vi "sig_processing.vi"(8 "error in (no error)":errorcluster, 9 "Operation":T1, 11 "Input Data Cluster":T3) -> (0 "error out":errorcluster, 3 "Output Data":T2)   [LabVIEW 2018]
uses:
  <vilib>/Utility/file.llb/Read Delimited Spreadsheet (string).vi
  <vilib>/Utility/file.llb/Read Delimited Spreadsheet (DBL).vi
  sig_processing_data_cluster.ctl
  sig_proc_output_data.ctl
  sig_processing_state_defining_enum.ctl
panel:
  out "Note":string
  in  "NotesPath":path
  in  "FreqsPath":path
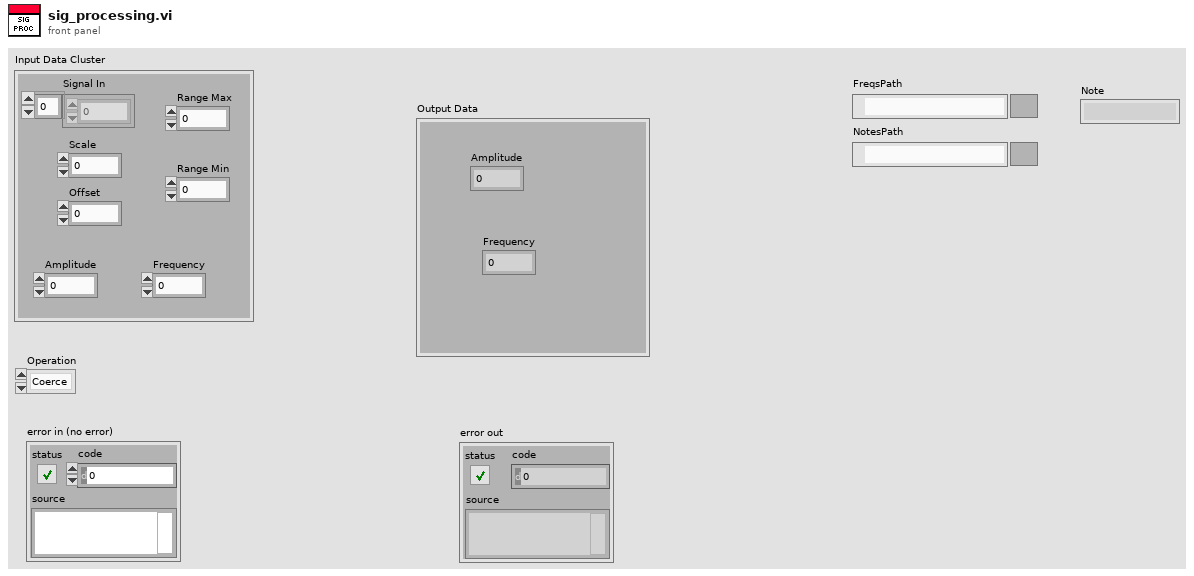
[diagram p1: front panel]
types:
  T1 = typedef "sig_processing_state_defining_enum.ctl" = enum16{"Coerce", "Scale", "Offset", "Norm"}
  T2 = typedef "sig_proc_output_data.ctl" = cluster{"Amplitude":dbl, "Frequency":dbl}
  T3 = typedef "sig_processing_data_cluster.ctl" = cluster{"Signal In":dbl[], "Scale":dbl, "Offset":dbl, "Range Max":dbl, "Range Min":dbl, "Amplitude":dbl, "Frequency":dbl}
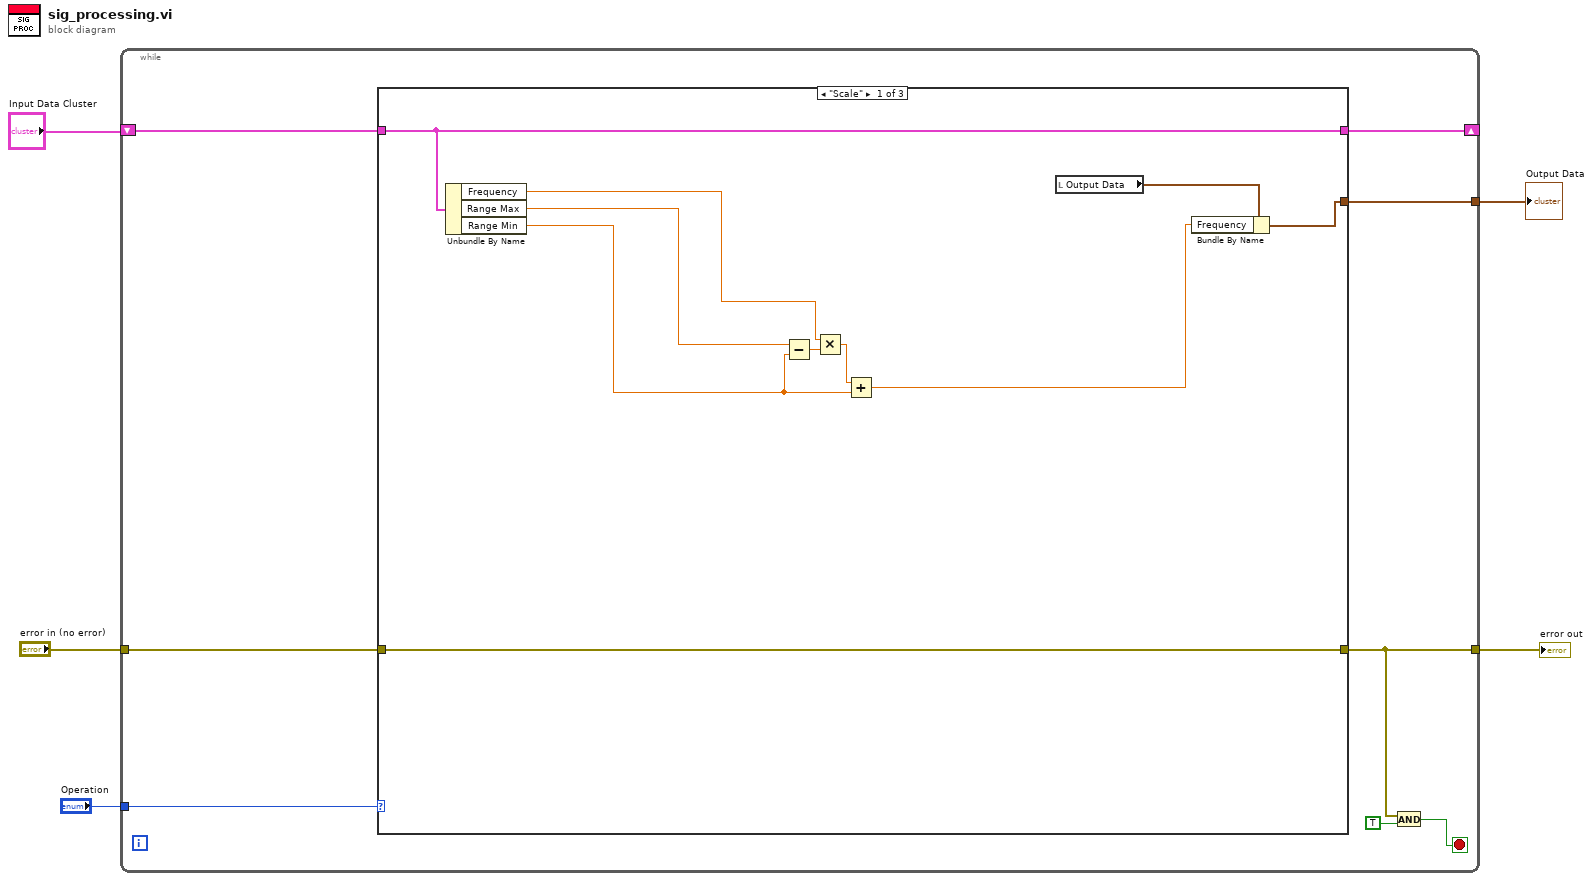
[diagram p0: block diagram]
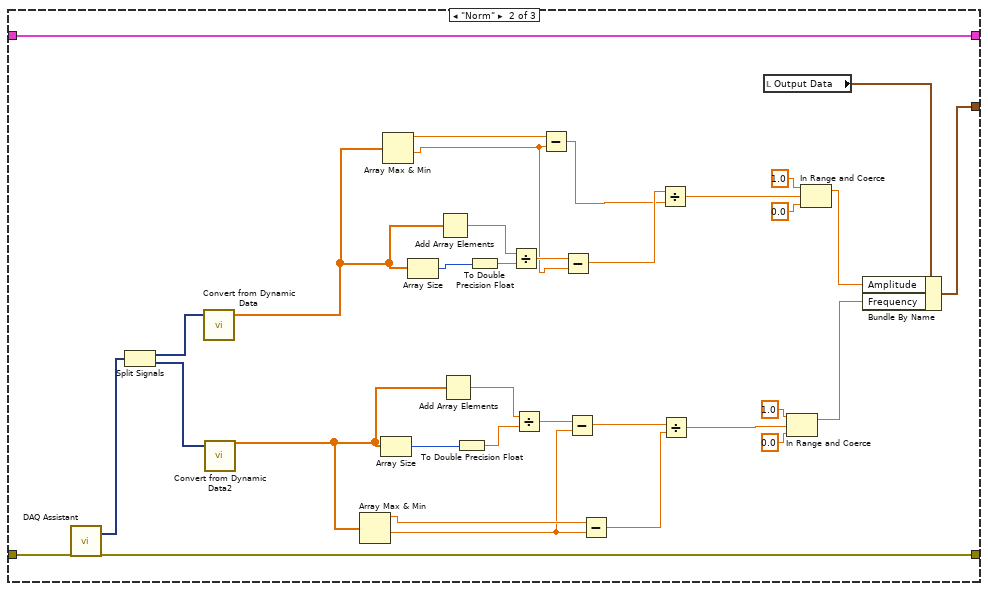
[diagram p2: hidden frame]
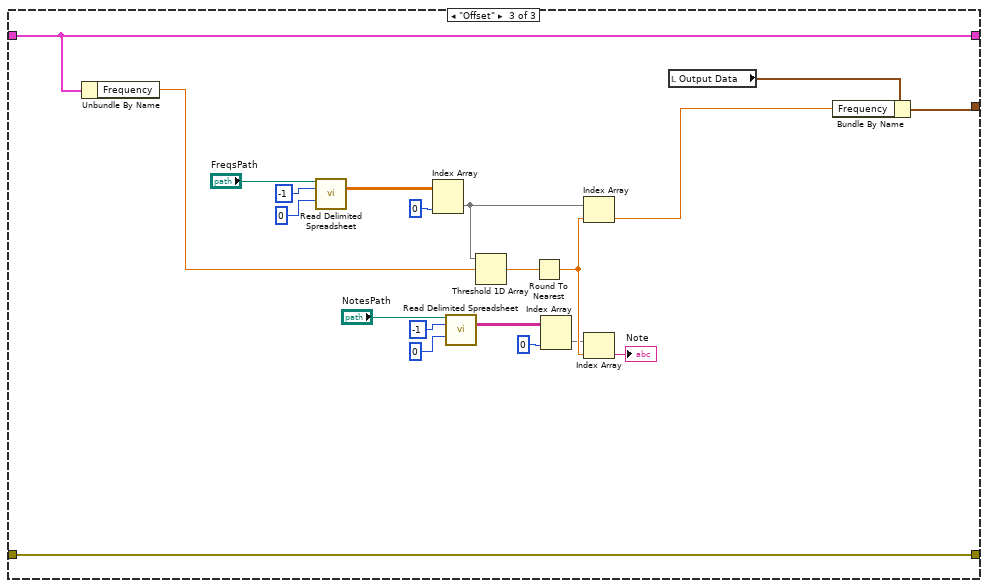
[diagram p3: hidden frame]
diagram:
  n1 = while {
    tunnel: "Operation" -> [w13]
    shift-right: [w10] -> _
    shift-left: "Input Data Cluster" -> [w11]
    tunnel: "error in (no error)" -> [w12]
    tunnel: [w8] -> w4
    tunnel: [w6] -> w2
    stop <- w7 stop-if-true
    n2 = case shown="\"Scale\"" w13 {
      tunnel: w12 -> [w23 w48 w78]
      tunnel: [w23 w47 w78] -> w8
      tunnel: w11 -> [w20 w42 w62]
      tunnel: [w20 w42 w62] -> w10
      tunnel: [w14 w33 w60] -> w6
      frame "Scale" {
        n3 = Unbundle By Name(w20) -> ("Frequency"=w19:dbl, "Range Max"=w18:dbl, "Range Min"=w17:dbl)
        n4 = Subtract(x=w18, y=w17) -> (x-y=w22:dbl)
        n5 = Multiply(x=w19, y=w22) -> (x*y=w21:dbl)
        n6 = Add(x=w21, y=w17) -> (x+y=w15:dbl)
        n7 = local read "Output Data"() -> (w16:T2)
        n8 = Bundle By Name(cluster=w16, "Frequency"=w15) -> (w14:T2)
      }
      frame "Norm" {
        n9 = call "DAQ Assistant"("error in"=w48) -> ("data"=w57:dynamicdata, "error out"=w47:errorcluster)  [unwired: 16 in, 1 out]
        n10 = Split Signals(w57) -> (w56:dynamicdata, w50:dynamicdata)  [unwired: 2 in]
        n11 = call "Convert from Dynamic Data"("Dynamic Data Type"=w56) -> ("Array"=w38:dbl[])  [unwired: 3 in]
        n12 = call "Convert from Dynamic Data2"("Dynamic Data Type"=w50) -> ("Array"=w37:dbl[])  [unwired: 3 in]
        n13 = Array Max & Min(array=w37) -> (max value=w36:dbl, min value=w34:dbl)  [unwired: 2 out]
        n14 = Array Size(array=w37) -> (size(s)=w51:i32)
        n15 = Array Max & Min(array=w38) -> (max value=w41:dbl, min value=w39:dbl)  [unwired: 2 out]
        n16 = Array Size(array=w38) -> (size(s)=w45:i32)
        n17 = Add Array Elements(numeric array=w38) -> (sum=w55:dbl)
        n18 = Add Array Elements(numeric array=w37) -> (sum=w52:dbl)
        n19 = To Double Precision Float(number=w51) -> (double precision float=w44:dbl)
        n20 = To Double Precision Float(number=w45) -> (double precision float=w46:dbl)
        n21 = Divide(x=w55, y=w46) -> (x/y=w54:dbl)
        n22 = Divide(x=w52, y=w44) -> (x/y=w49:dbl)
        n23 = Subtract(x=w41, y=w39) -> (x-y=w40:dbl)
        n24 = Subtract(x=w54, y=w39) -> (x-y=w53:dbl)
        n25 = Subtract(x=w49, y=w34) -> (x-y=w43:dbl)
        n26 = Subtract(x=w36, y=w34) -> (x-y=w35:dbl)
        n27 = Divide(x=w53, y=w40) -> (x/y=w25:dbl)
        n28 = Divide(x=w43, y=w35) -> (x/y=w29:dbl)
        n29 = local read "Output Data"() -> (w32:T2)
        n30 = In Range and Coerce(upper limit=1.0, x=w29, lower limit=0.0) -> (coerced(x)=w28:dbl)  [unwired: 1 out]
        n31 = In Range and Coerce(upper limit=1.0, x=w25, lower limit=0.0) -> (coerced(x)=w24:dbl)  [unwired: 1 out]
        n32 = Bundle By Name(cluster=w32, "Amplitude"=w24, "Frequency"=w28) -> (w33:T2)
      }
      frame "Offset" {
        n33 = Unbundle By Name(w62) -> ("Frequency"=w61:dbl)
        n34 = call-poly <vilib>:"Read Delimited Spreadsheet.vi"("file path (dialog if empty)"="FreqsPath", "number of rows (all:-1)"=-1, "max characters/row  (no limit:0)"=0) -> ("all rows"=w74:dbl[][])  [unwired: 7 in, 5 out]
        n35 = Index Array(array=w74, index (col)=0 ("index (row)")) -> (element=w66:dbl[])  [unwired: 1 in]
        n36 = call-poly <vilib>:"Read Delimited Spreadsheet.vi"("file path (dialog if empty)"="NotesPath", "number of rows (all:-1)"=-1, "max characters/row  (no limit:0)"=0) -> ("all rows"=w69:string[][])  [unwired: 7 in, 5 out]
        n37 = Threshold 1D Array(2:w61, 3:w66) -> (0:w67:dbl)  [unwired: 1 in]
        n38 = Round To Nearest(number=w67) -> (nearest integer value=w65:dbl)
        n39 = Index Array(array=w69, index (col)=0 ("index (row)")) -> (element=w64:string[])  [unwired: 1 in]
        n40 = Index Array(array=w66, index=w65) -> (element=w58:dbl)
        n41 = Index Array(array=w64, index=w65) -> (element=→"Note":string)
        n42 = local read "Output Data"() -> (w59:T2)
        n43 = Bundle By Name(cluster=w59, "Frequency"=w58) -> (w60:T2)
      }
    }
    n44 = And(x=w8, y=TRUE) -> (x .and. y?=w7:bool)
  }
  "error out" <- w4
  "Output Data" <- w2
